vi "Process Multi-LineState String.vi"(11 "Multi-line State String":string) -> (3 "State Array":string[](array[string]))   [LabVIEW 2023]
uses:
  <userlib>/_OpenG.lib/string/string.llb/openg_string.lvlib
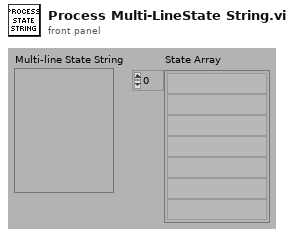
[diagram p1: front panel]
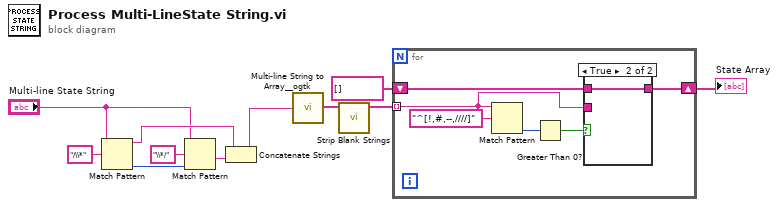
[diagram p0: block diagram]
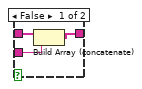
[diagram p2: hidden frame]
diagram:
  n1 = Match Pattern(string="Multi-line State String", regular expression="/\\*") -> (before substring=w7:string, offset past match=w9:i32)  [unwired: 1 in, 2 out]
  n2 = Match Pattern(string="Multi-line State String", regular expression="\\*/", offset (0)=w9) -> (after substring=w6:string)  [unwired: 3 out]
  n3 = Concatenate Strings(w7, w6) -> (w4:string)
  n4 = call <userlib>:"Multi-line String to Array__ogtk.vi"("string"=w4) -> ("lines"=w11:string[])
  n5 = call "Strip Blank Strings.vi"("ArrayIn"=w11) -> ("Array Out"=w3:string[])  [unwired: 10 in]
  n6 = for {
    tunnel: w3 -> [w13] mode=indexing
    shift-right: [w12] -> w1
    shift-left: string[] [] -> [w14]
    n7 = Match Pattern(string=w13, regular expression="^[!,#,--,////]") -> (offset past match=w16:i32)  [unwired: 1 in, 3 out]
    n8 = Greater Than 0?(x=w16) -> (x > 0?=w15:bool)
    n9 = case shown="True" w15 {
      tunnel: w14 -> [w20 w21]
      tunnel: w13 -> [w19 _]
      tunnel: [w18 w21] -> w12
      frame False {
        n10 = Build Array (concatenate)(w20, w19) -> (w18:string[])
      }
      frame True {
      }
    }
  }
  "State Array" <- w1
